vi "Stop Core.vi"(10 "final error code":i32, 11 "DIMDemoClient in":refnum<class "DIMDemoClient.lvclass">) -> (3 "DIMDemoClient out":refnum<class "DIMDemoClient.lvclass">)   [LabVIEW 2012, in "DimActorDemo.lvlib" / "DIMDemoClient.lvclass"]
doc: "Release DIM services, commands and subscribtions."
uses:
  DIMDemoClient.lvclass
  DIMActor/DIMActor/DIMActor.lvclass
  DIMDemoClient.lvclass/DIMDemoClient.ctl
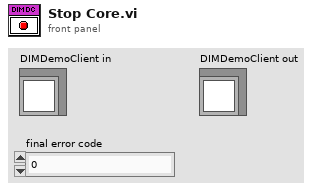
[diagram p1: front panel]
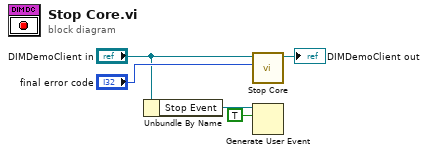
[diagram p0: block diagram]
diagram:
  n1 = Unbundle By Name("DIMDemoClient in") -> ("Stop Event"=w2:refnum<user-event>)
  n2 = call-parent "Stop Core.vi"("final error code"="final error code", "DIMActor in"="DIMDemoClient in") -> ("DIMActor out"=→"DIMDemoClient out":refnum<class "DIMDemoClient.lvclass">)  [unwired: 9 in]
  n3 = Generate User Event(user event=w2, event data cluster=TRUE ("event data")) -> ()  [unwired: 1 in, 2 out]
